vi "Email_List_subvi.vi"(8 "Open File":bool, 9 "Name Ring In":u16(ring) items=["Jeremy", "Pete"], 10 "List Location":path, 11 "Text Editor Location":path) -> (0 "String":string, 1 "Names Out":string[](array[string]), 3 "Open File Clear":bool)   [LabVIEW 2012]
uses:
  <vilib>/Utility/file.llb/Write To Spreadsheet File (string).vi
  <vilib>/Utility/file.llb/Read From Spreadsheet File (string).vi
panel:
  in  "command line 1":string="notepad LabVIEW.ini"
  out "Array":string[][](array[string])
  out "Name Ring Out":u16(ring) items=["Chris", "Derek", "Jeremy", "Joshua", "Katelyn", "Loah", "Oana", "Pete"]
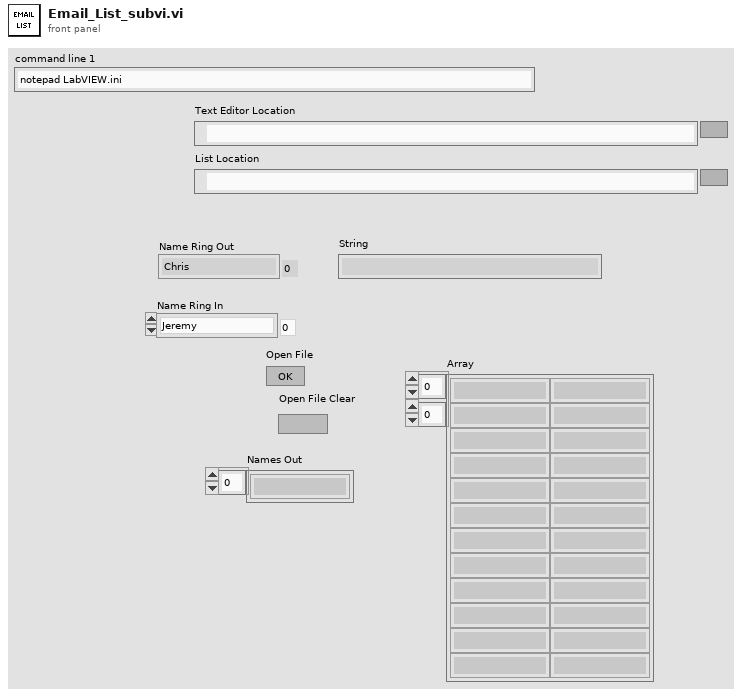
[diagram p1: front panel]
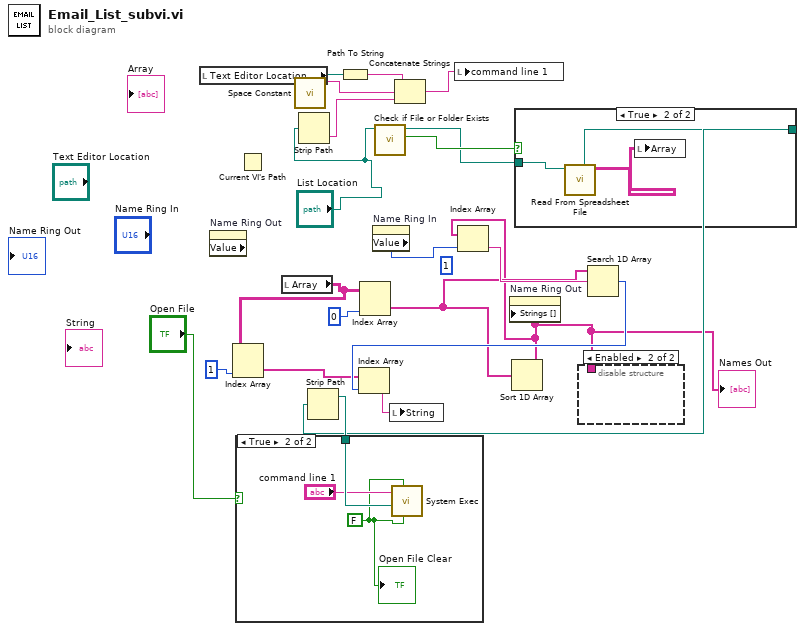
[diagram p0: block diagram]
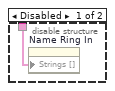
[diagram p2: hidden frame]
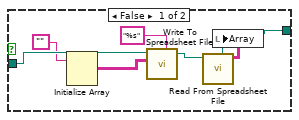
[diagram p4: hidden frame]
diagram:
  (unwired) 1
  n1 = local read "Text Editor Location"() -> (w10:path)
  n2 = property on="Name Ring Out" class="Ring (strict)" props=["Value"]() -> ()  [unwired: 2 in, 3 out]
  n3 = Current VI's Path() -> ()  [unwired: 1 out]
  n4 = local read "Array"() -> (w14:string[][])
  n5 = Index Array(array=w14, index (col)=1) -> (element=w12:string[])  [unwired: 1 in]
  n6 = call <vilib>:"Space Constant.vi"() -> ("String"=w6:string)
  n7 = Strip Path(path="List Location") -> (name=w7:string)  [unwired: 1 out]
  n8 = Path To String(path=w10) -> (string=w9:string)
  n9 = Index Array(array=w14, index (col)=0) -> (element=w15:string[])  [unwired: 1 in]
  n10 = property on="Name Ring In" class="Ring (strict)"() -> ("Value"=w2:u16)  [unwired: 2 in, 2 out]
  n11 = call <vilib>:"Check if File or Folder Exists.vi"("path"="List Location") -> ("file or folder exists?"=w21:bool, "dup path"=w20:path)  [unwired: 8 in, 1 out]
  n12 = Concatenate Strings(w9, w6, w7) -> (w5:string)
  n13 = local write "command line 1"(w5) -> ()
  n14 = Sort 1D Array(array=w15) -> (sorted array=w1:string[])
  "Names Out" <- w1
  n15 = Index Array(array=w1, index=w2) -> (element=w18:string)
  n16 = property on="Name Ring Out" class="Ring (strict)"("Strings []"=w1) -> ()  [unwired: 2 in, 2 out]
  n17 = case shown="True" w21 {
    tunnel: w20 -> [w28 w31]
    tunnel: [w24 w29] -> w4
    frame False {
      n18 = Initialize Array("") -> (w22:string[][])  [unwired: 2 in]
      n19 = call-poly <vilib>:"Write To Spreadsheet File.vi"("format (%s)"="%s", "2D data"=w22, "file path (dialog if empty)"=w28) -> ("new file path (Not A Path if cancelled)"=w27:path)  [unwired: 5 in]
      n20 = call-poly <vilib>:"Read From Spreadsheet File.vi"("file path (dialog if empty)"=w27) -> ("all rows"=w25:string[][], "new file path (Not A Path if cancelled)"=w24:path)  [unwired: 6 in, 3 out]
      n21 = local write "Array"(w25) -> ()
    }
    frame True {
      n22 = call-poly <vilib>:"Read From Spreadsheet File.vi"("file path (dialog if empty)"=w31) -> ("all rows"=w30:string[][], "new file path (Not A Path if cancelled)"=w29:path)  [unwired: 6 in, 3 out]
      n23 = local write "Array"(w30) -> ()
    }
  }
  n24 = Strip Path(path=w4) -> (stripped path=w11:path)  [unwired: 1 out]
  n25 = case shown="True" "Open File" {
    tunnel: w11 -> [_ w34]
    frame False {
    }
    frame True {
      w32 = FALSE
      n26 = call <vilib>:"System Exec.vi"("run minimized? (F)"=w32, "wait until completion? (T)"=w32, "working directory"=w34, "command line"="command line 1") -> ()  [unwired: 2 in, 6 out]
      "Open File Clear" <- w32
    }
  }
  n27 = disable-structure shown="Enabled" {
    disable-tunnel: w1 -> [w35 _]
    frame Disabled {
      n28 = property on="Name Ring In" class="Ring (strict)"("Strings []"=w35) -> ()  [unwired: 2 in, 2 out]
    }
    frame Enabled {
    }
  }
  n29 = Search 1D Array(1D array=w15, element=w18) -> (index of element=w16:i32)  [unwired: 1 in]
  n30 = Index Array(array=w12, index=w16) -> (element=w17:string)
  n31 = local write "String"(w17) -> ()
